vi "Queue Manager.vi"(7 "Task":T3=enum."Send", 8 "error in":errorcluster, 10 "Command":T1) -> (0 "error out":errorcluster, 3 "Queue":refnum<queue>)   [LabVIEW 2019, in "ASCII Actor.lvlib"]
doc: "Template for managing a queue. The Dequeue operations should be done outside of this VI since a queue should be a one-read-many-write paradigm."
uses:
  ASCII Actor.lvlib
  Queue Task.ctl
  Actor Command.ctl
  Actor Task.ctl
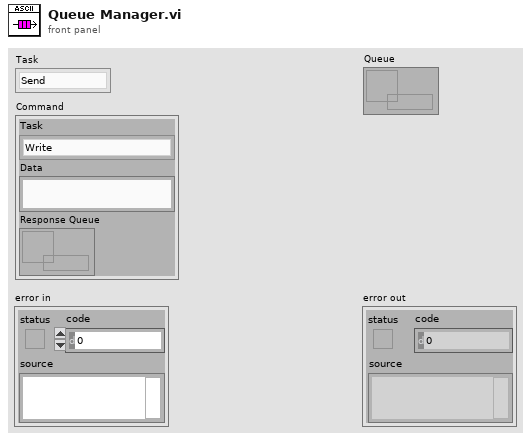
[diagram p1: front panel]
types:
  T1 = typedef "ASCII Actor.lvlib/Actor Command.ctl" = cluster{"Task":T2, "Data":string, "Response Queue":refnum<queue>}
  T2 = typedef "ASCII Actor.lvlib/Actor Task.ctl" = enum8{"Write", "Get Data", "Stop"}
  T3 = typedef "ASCII Actor.lvlib/Queue Task.ctl" = enum8{"Get Reference", "Send", "Close"}
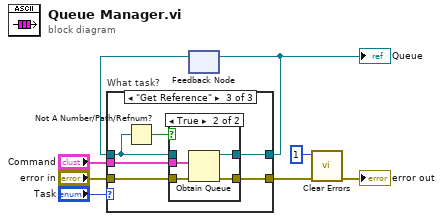
[diagram p0: block diagram]
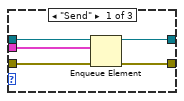
[diagram p2: hidden frame]
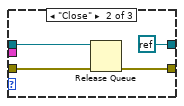
[diagram p3: hidden frame]
diagram:
  n1 = feedback #1() -> (w4:refnum<queue>)  [unwired: 1 out]
  n2 = case "What task?" shown="\"Get Reference\"" "Task" {
    tunnel: "error in" -> [w13 w17 w23]
    tunnel: [w12 w16 w22] -> w7
    tunnel: [w10 refnum<k0> refnum w21] -> w5
    tunnel: w4 -> [w11 w15 w19]
    tunnel: "Command" -> [w9 _ w20]
    frame "Send" {
      n3 = Enqueue Element(queue=w11, element=w9, error in (no error)=w13) -> (queue out=w10:refnum<queue>, error out=w12:errorcluster)  [unwired: 2 out]
    }
    frame "Close" {
      n4 = Release Queue(queue=w15, error in (no error)=w17) -> (error out=w16:errorcluster)  [unwired: 1 in, 2 out]
    }
    frame "Get Reference" {
      n5 = Not A Number/Path/Refnum?(number/path/refnum=w19) -> (NaN/Path/Refnum?=w18:bool)
      n6 = case shown="True" w18 {
        tunnel: w23 -> [w25 w29]
        tunnel: [w25 w28] -> w22
        tunnel: [w24 w27] -> w21
        tunnel: w20 -> [_ w26]
        tunnel: w19 -> [w24 _]
        frame False {
        }
        frame True {
          n7 = Obtain Queue(element data type=w26, error in (no error)=w29) -> (queue out=w27:refnum<queue>, error out=w28:errorcluster)  [unwired: 2 in, 2 out]
        }
      }
    }
  }
  "Queue" <- w5
  n8 = feedback-in #1(w5) -> ()
  n9 = call <vilib>:"Clear Errors.vi"("error in (no error)"=w7, "specific error code to clear (0: all)"=1 ("Clear All?")) -> ("error out"=→"error out":errorcluster)  [unwired: 4 in, 1 out]
